vi "ArrayOperations.vi"() -> ()   [LabVIEW 2015]
panel:
  in  "index 2":i32
  out "second subarray":dbl[](array[numeric])
  out "first subarray":dbl[](array[numeric])
  out "x+y":dbl[](array[numeric])
  out "subarray":dbl[](array[numeric])
  in  "length":i32
  in  "index":i32
  out "element":dbl
  out "index of element":i32
  in  "Buscador":dbl
  out "min":dbl
  out "max":dbl
  out "Arreglo Ordenado\nAscendentemente":dbl[](array[numeric])
  out "Arreglo\nInvertido":dbl[](array[numeric])
  out "Arreglo\nFinal":dbl[](array[numeric])
  in  "Factor de\nEscala":dbl
  out "Arreglo\nAleatorio":dbl[](array[numeric])
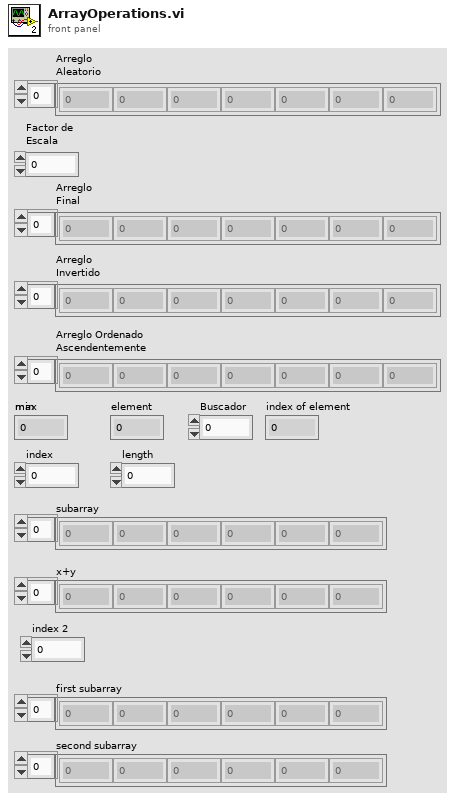
[diagram p1: front panel]
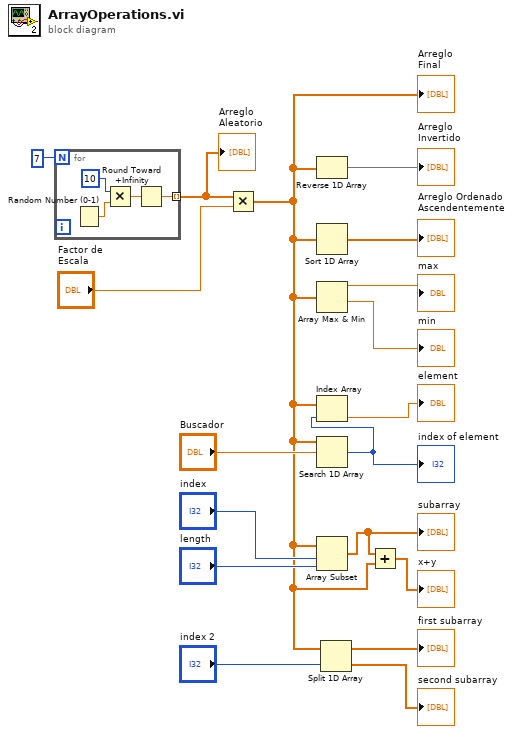
[diagram p0: block diagram]
diagram:
  n1 = for {
    N: 7 -> [_]
    tunnel: [w19] -> w17 mode=indexing
    n2 = Random Number (0-1)() -> (number: 0 to 1=w21:dbl)
    n3 = Multiply(x=10, y=w21) -> (x*y=w20:dbl)
    n4 = Round Toward +Infinity(x=w20) -> (ceil(x): smallest int >= x=w19:dbl)
  }
  "Arreglo\nAleatorio" <- w17
  n5 = Multiply(x=w17, y="Factor de\nEscala") -> (x*y=w4:dbl[])
  "Arreglo\nFinal" <- w4
  n6 = Reverse 1D Array(array=w4) -> (reversed array=→"Arreglo\nInvertido":dbl[])
  n7 = Sort 1D Array(array=w4) -> (sorted array=→"Arreglo Ordenado\nAscendentemente":dbl[])
  n8 = Array Max & Min(array=w4) -> (max value=→"max":dbl, min value=→"min":dbl)  [unwired: 2 out]
  n9 = Search 1D Array(1D array=w4, element="Buscador") -> (index of element=w10:i32)  [unwired: 1 in]
  "index of element" <- w10
  n10 = Index Array(array=w4, index=w10) -> (element=→"element":dbl)
  n11 = Array Subset(array=w4, index="index", length="length") -> (w6:dbl[])
  "subarray" <- w6
  n12 = Split 1D Array(array=w4, index="index 2") -> (first subarray=→"first subarray":dbl[], second subarray=→"second subarray":dbl[])
  n13 = Add(x=w6, y=w4) -> (x+y=→"x+y":dbl[])
